vi "example test.vi"() -> ()   [LabVIEW 2013, in "OPC UA Client Tests.lvlib"]
uses:
  OPC UA Client Tests.lvlib
  module/configuration/OPC UA Client configuration.lvclass
  <vilib>/NI/Tag Bus Module Framework/channel/TBM channel.lvclass
  <vilib>/NI/Tag Bus/tag/Data Type.ctl
  <vilib>/NI/Tag Bus/tag/tag descriptor.lvclass
  <vilib>/NI/Tag Bus Module Framework/channel/channel classification.ctl
  module/execution/OPC UA runtime.lvclass
  <vilib>/NI/Tag Bus/dictionary/data dictionary.lvclass
  <vilib>/NI/Tag Bus/dictionary/lookup polymorphs/locate double.vi
  <vilib>/NI/Tag Bus/table/data table.lvlib
  <vilib>/NI/Tag Bus/table/data polymorphs/write one/write Double.vi
  <vilib>/NI/Configuration Framework/serializable configuration/NISE_CEF_serializable configuration.lvclass
  <vilib>/NI/Tag Bus/table/data polymorphs/read one/read Double.vi
panel:
  out "final error":errorcluster
  out "output error":errorcluster
  out "input error":errorcluster
  out "output lookup error":errorcluster
  out "no data written":bool
  out "input lookup error":errorcluster
  out "init error":errorcluster
  out "correct execution settings":bool
  out "serialization problem":errorcluster
  out "invalid configuration":errorcluster
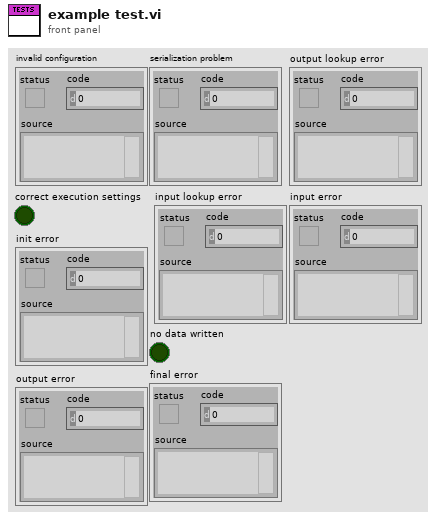
[diagram p1: front panel]
types:
  T1 = typedef "TBM channel.lvclass/channel classification.ctl" = enum16{"input data", "output data", "processing parameter", "processing result"}
  T2 = typedef "tag bus.lvlib/tag descriptor.lvclass/Data Type.ctl" = enum16{"Double", "Single", "I64", "I32", "I16", "I8", "U64", "U32", "U16", "U8", "Boolean", "String", "Array of Double", "Array of Single", "Array of I64", "Array of I32", "Array of I16", "Array of I8", "Array of U64", "Array of U32", "Array of U16", "Array of U8", "Array of Boolean", "Array of String"}
  T3 = cluster{"channel":refnum<class "TBM channel.lvclass">}
  T4 = typedef "TBM channel.lvclass/data tables.ctl" = cluster{"input data":T5, "processing parameter":T5, "processing result":T5, "output data":T5}
  T5 = typedef "tag bus.lvlib/dictionary table pair.ctl" = cluster{"data dictionary":refnum<class "data dictionary.lvclass">, "data table":T6}
  T6 = typedef "tag bus.lvlib/data table.lvlib/data table.ctl" = cluster{"Double":dbl[], "Single":sgl[], "I64":i64[], "I32":i32[], "I16":i16[], "I8":i8[], "U64":u64[], "U32":u32[], "U16":u16[], "U8":u8[], "Boolean":bool[], "String":string[], "Array of Double":cluster{"DBL Array":dbl[]}[], "Array of Single":cluster{"SGL Array":sgl[]}[], "Array of I64":cluster{"I64 Array":i64[]}[], "Array of I32":cluster{"I32 Array":i32[]}[], "Array of I16":cluster{"I16 Array":i16[]}[], "Array of I8":cluster{"I8 Array":i8[]}[], "Array of U64":cluster{"U64 Array":u64[]}[], "Array of U32":cluster{"U32 Array":u32[]}[], "Array of U16":cluster{"U16 Array":u16[]}[], "Array of U8":cluster{"U8 Array":u8[]}[], "Array of Boolean":cluster{"Boolean Array":bool[]}[], "Array of String":cluster{"String Array":string[]}[]}
  T7 = typedef "TBM module execution interface.lvclass/execution settings.ctl" = cluster{"reads inputs":bool, "processes data":bool, "writes outputs":bool}
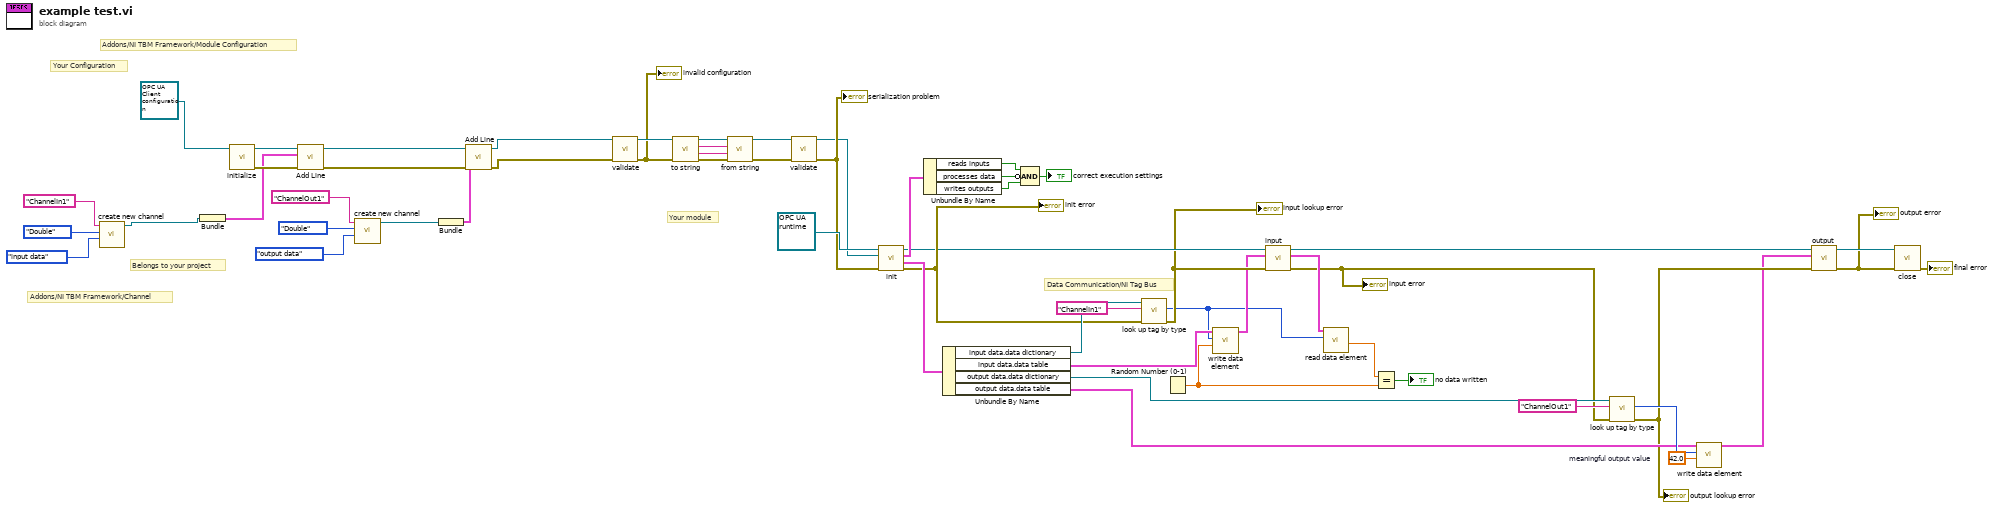
[diagram p0: block diagram]
diagram:
  w18 = 42.0  # meaningful output value
  # "Data Communication/NI Tag Bus"
  # "Your module"
  # "Your Configuration"
  # "Addons/NI TBM Framework/Module Configuration"
  # "Belongs to your project"
  # "Addons/NI TBM Framework/Channel"
  n1 = call <vilib>:"create new channel.vi"("channel classification"=channel_classification."input data", "data type"=Data_Type."Double", "channel name"="ChannelIn1") -> ("channel"=w4:refnum<class "TBM channel.lvclass">)  [unwired: 8 in]
  n2 = Bundle("channel"=w4) -> (w3:T3)  [unwired: 1 in]
  n3 = call <vilib>:"initialize.vi"("configuration in"=refnum<class "OPC UA Client configuration.lvclass"> refnum ("tag bus configurable plugin module configuration")) -> ("error out"=w6:errorcluster, "configuration out"=w7:refnum<class "OPC UA Client configuration.lvclass">)  [unwired: 8 in, 1 out]
  n4 = call "Add Line.vi"("error in"=w6, "Line"=w3, "OPC UA configuration in"=w7) -> ("error out"=w8:errorcluster, "OPC UA configuration out"=w10:refnum<class "OPC UA Client configuration.lvclass">)  [unwired: 7 in]
  n5 = call <vilib>:"create new channel.vi"("channel classification"=channel_classification."output data", "data type"=Data_Type."Double", "channel name"="ChannelOut1") -> ("channel"=w2:refnum<class "TBM channel.lvclass">)  [unwired: 8 in]
  n6 = Bundle("channel"=w2) -> (w1:T3)  [unwired: 1 in]
  n7 = call "Add Line.vi"("error in"=w8, "Line"=w1, "OPC UA configuration in"=w10) -> ("error out"=w5:errorcluster, "OPC UA configuration out"=w9:refnum<class "OPC UA Client configuration.lvclass">)  [unwired: 7 in]
  n8 = call-dynamic "validate.vi"("error in"=w5, "OPC UA configuration in"=w9) -> ("error out"=w51:errorcluster, "OPC UA configuration out"=w52:refnum<class "OPC UA Client configuration.lvclass">)  [unwired: 8 in]
  "invalid configuration" <- w51
  n9 = call-dynamic "to string.vi"("error in"=w51, "OPC UA configuration in"=w52) -> ("error out"=w47:errorcluster, "data"=w48:string, "version"=w49:string, "OPC UA configuration out"=w50:refnum<class "OPC UA Client configuration.lvclass">)  [unwired: 6 in]
  n10 = call-dynamic "from string.vi"("error in"=w47, "data"=w48, "version"=w49, "OPC UA configuration in"=w50) -> ("error out"=w45:errorcluster, "OPC UA configuration out"=w46:refnum<class "OPC UA Client configuration.lvclass">)  [unwired: 6 in]
  n11 = call-dynamic "validate.vi"("error in"=w45, "OPC UA configuration in"=w46) -> ("error out"=w43:errorcluster, "OPC UA configuration out"=w42:refnum<class "OPC UA Client configuration.lvclass">)  [unwired: 8 in]
  "serialization problem" <- w43
  n12 = call-dynamic "init.vi"("error in"=w43, "TBM module configuration in"=w42, "OPC UA runtime in"=refnum<class "OPC UA runtime.lvclass"> refnum ("tag bus configurable plugin module")) -> ("error out"=w34:errorcluster, "data allocations"=w36:T4, "execution settings"=w41:T7, "OPC UA runtime out"=w31:refnum<class "OPC UA runtime.lvclass">)  [unwired: 5 in]
  "init error" <- w34
  n13 = Unbundle By Name(w41) -> ("reads inputs"=w38:bool, "processes data"=w40:bool, "writes outputs"=w39:bool)
  n14 = Unbundle By Name(w36) -> ("input data.data dictionary"=w35:refnum<class "data dictionary.lvclass">, "input data.data table"=w32:T6, "output data.data dictionary"=w23:refnum<class "data dictionary.lvclass">, "output data.data table"=w20:T6)
  n15 = Compound Arithmetic op=AND(w38, invert w40, w39) -> (→"correct execution settings":bool)
  n16 = call-poly <vilib>:"look up tag by type.vi"("error in"=w34, "name"="ChannelIn1" ("channel name"), "data dictionary in"=w35) -> ("error out"=w30:errorcluster, "index"=w27:i32)  [unwired: 6 in, 1 out]
  "input lookup error" <- w30
  n17 = Random Number (0-1)() -> (number: 0 to 1=w26:dbl)
  n18 = call-poly <vilib>:"write data element.vi"("value"=w26, "index"=w27, "data table in"=w32) -> ("data table out"=w29:T6)  [unwired: 8 in]
  n19 = call-dynamic "input.vi"("error in"=w30, "data table in"=w29, "OPC UA runtime in"=w31) -> ("error out"=w19:errorcluster, "data table out"=w28:T6, "OPC UA runtime out"=w16:refnum<class "OPC UA runtime.lvclass">)  [unwired: 6 in]
  "input error" <- w19
  n20 = call-poly <vilib>:"read data element.vi"("index"=w27, "data table in"=w28) -> ("value"=w25:dbl)  [unwired: 8 in, 1 out]
  n21 = Equal?(x=w25, y=w26) -> (x = y?=→"no data written":bool)
  n22 = call-poly <vilib>:"look up tag by type.vi"("error in"=w19, "name"="ChannelOut1" ("channel name"), "data dictionary in"=w23) -> ("error out"=w17:errorcluster, "index"=w21:i32)  [unwired: 6 in, 1 out]
  "output lookup error" <- w17
  n23 = call-poly <vilib>:"write data element.vi"("value"=w18, "index"=w21, "data table in"=w20) -> ("data table out"=w15:T6)  [unwired: 8 in]
  n24 = call-dynamic "output.vi"("error in"=w17, "data table in"=w15, "OPC UA runtime in"=w16) -> ("error out"=w13:errorcluster, "OPC UA runtime out"=w14:refnum<class "OPC UA runtime.lvclass">)  [unwired: 6 in, 1 out]
  "output error" <- w13
  n25 = call-dynamic "close.vi"("error in"=w13, "OPC UA runtime in"=w14) -> ("error out"=→"final error":errorcluster)  [unwired: 9 in]
